vi "ABR-Analyze.vi"(0 "Neural (uV)":dbl[](array[numeric]), 2 "Runtime":T1, 5 "microphonic (uV)":dbl[](array[numeric]), 7 "Averaging data":cluster{i32, i32}, 9 "Normalize individual?":bool, 11 "error in":errorcluster, 12 "Analysis":T3, 13 "Graphs":T2) -> (4 "spread value":dbl, 14 "Analysis out":T3, 15 "error out":errorcluster)   [LabVIEW 2020]
uses:
  TypeDefs/ABR-Analysis State.ctl
  Threshold Estimation VIs/ABR3-Threshold Estimation Result.ctl
  TypeDefs/ABR3-Graph Controls.ctl
  TypeDefs/ABR-Runtime Data.ctl
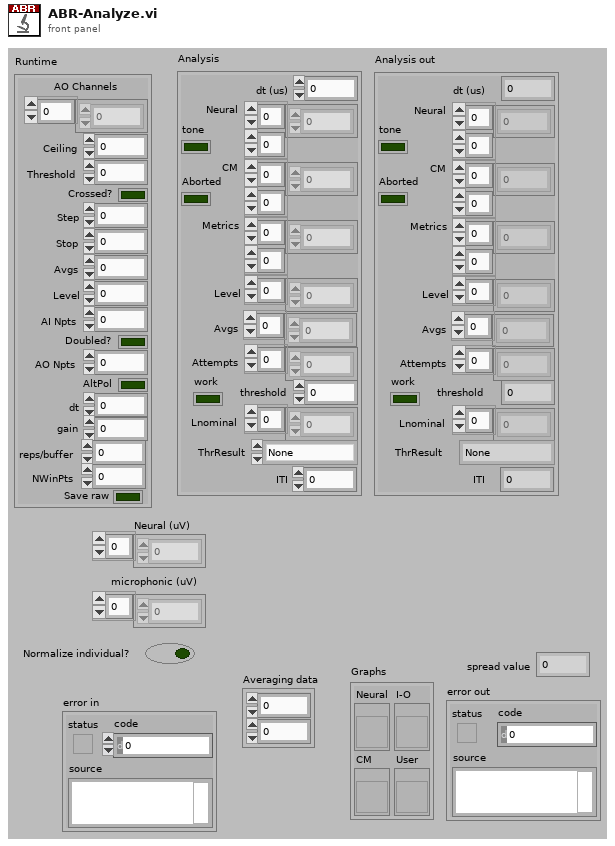
[diagram p1: front panel]
types:
  T1 = typedef "ABR-Runtime Data.ctl" = cluster{"AO Channels":i32[], "Ceiling":dbl, "Threshold":dbl, "Crossed?":bool, "Step":dbl, "Stop":i32, "Avgs":i32, "Level":dbl, "AI Npts":i32, "Doubled?":bool, "AO Npts":i32, "AltPol":bool, "dt":dbl, "gain":dbl, "reps/buffer":i32, "NWinPts":i32, "Save raw":bool}
  T2 = typedef "ABR3-Graph Controls.ctl" = cluster{"I-O":refnum<vi>, "Neural":refnum<vi>, "CM":refnum<vi>, "User":refnum<vi>}
  T3 = typedef "ABR-Analysis State.ctl" = cluster{"dt (us)":dbl, "Neural":dbl[][], "CM":dbl[][], "Metrics":dbl[][], "Level":dbl[], "Avgs":i32[], "Attempts":i32[], "Aborted":bool, "threshold":dbl, "Lnominal":dbl[], "tone":bool, "work":bool, "ThrResult":T4, "ITI":dbl}
  T4 = typedef "ABR3-Threshold Estimation Result.ctl" = enum16{"None", "Power", "Sigmoid", "Power (noisy)", "Suprathreshold", "Invalid"}
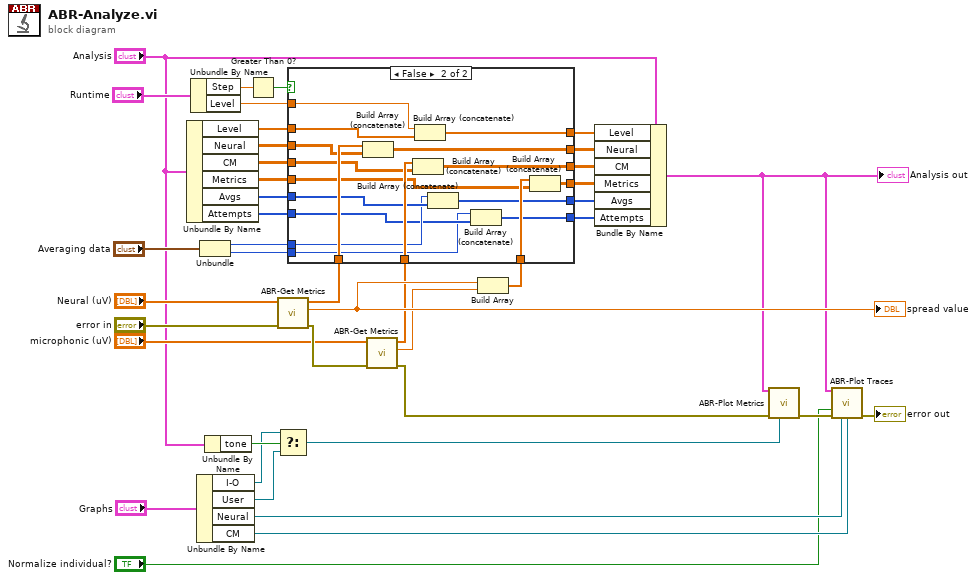
[diagram p0: block diagram]
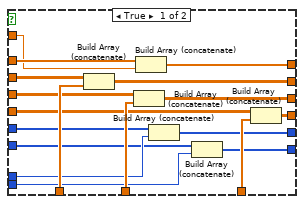
[diagram p2: hidden frame]
diagram:
  n1 = Unbundle By Name("Analysis") -> ("Level"=w27:dbl[], "Neural"=w35:dbl[][], "CM"=w34:dbl[][], "Metrics"=w33:dbl[][], "Avgs"=w18:i32[], "Attempts"=w14:i32[])
  n2 = Unbundle By Name("Runtime") -> ("Step"=w2:dbl, "Level"=w25:dbl)
  n3 = Unbundle By Name("Graphs") -> ("I-O"=w5:refnum<vi>, "User"=w4:refnum<vi>, "Neural"=w21:refnum<vi>, "CM"=w20:refnum<vi>)
  n4 = Unbundle("Averaging data") -> (w16:i32, w12:i32)
  n5 = Unbundle By Name("Analysis") -> ("tone"=w6:bool)
  n6 = Greater Than 0?(x=w2) -> (x > 0?=w1:bool)
  n7 = call "ABR-Get Metrics.vi"("error in (no error)"="error in", "Data in"="Neural (uV)") -> ("error out"=w29:errorcluster, "spread value"=w41:dbl, "Data out"=w39:dbl[])  [unwired: 7 in]
  "spread value" <- w41
  n8 = Select(t=w5, s=w6, f=w4) -> (s? t:f=w3:refnum<vi>)
  n9 = call "ABR-Get Metrics.vi"("error in (no error)"=w29, "Data in"="microphonic (uV)") -> ("error out"=w11:errorcluster, "spread value"=w37:dbl, "Data out"=w38:dbl[])  [unwired: 7 in]
  n10 = Build Array(w41, w37) -> (w40:dbl[])
  n11 = case shown="False" w1 {
    tunnel: w40 -> [w59 w77]
    tunnel: w39 -> [w58 w76]
    tunnel: w38 -> [w57 w75]
    tunnel: w35 -> [w56 w74]
    tunnel: w34 -> [w55 w73]
    tunnel: w33 -> [w54 w72]
    tunnel: [w53 w71] -> w32
    tunnel: [w52 w70] -> w31
    tunnel: [w51 w69] -> w30
    tunnel: w27 -> [w50 w68]
    tunnel: [w49 w67] -> w26
    tunnel: w25 -> [w48 w66]
    tunnel: w18 -> [w47 w65]
    tunnel: w16 -> [w46 w64]
    tunnel: [w45 w63] -> w15
    tunnel: w14 -> [w44 w62]
    tunnel: [w43 w61] -> w13
    tunnel: w12 -> [w42 w60]
    frame True {
      n12 = Build Array (concatenate)(w56, w58) -> (w53:dbl[][])
      n13 = Build Array (concatenate)(w55, w57) -> (w52:dbl[][])
      n14 = Build Array (concatenate)(w50, w48) -> (w49:dbl[])
      n15 = Build Array (concatenate)(w47, w46) -> (w45:i32[])
      n16 = Build Array (concatenate)(w44, w42) -> (w43:i32[])
      n17 = Build Array (concatenate)(w54, w59) -> (w51:dbl[][])
    }
    frame False {
      n18 = Build Array (concatenate)(w76, w74) -> (w71:dbl[][])
      n19 = Build Array (concatenate)(w75, w73) -> (w70:dbl[][])
      n20 = Build Array (concatenate)(w66, w68) -> (w67:dbl[])
      n21 = Build Array (concatenate)(w64, w65) -> (w63:i32[])
      n22 = Build Array (concatenate)(w60, w62) -> (w61:i32[])
      n23 = Build Array (concatenate)(w77, w72) -> (w69:dbl[][])
    }
  }
  n24 = Bundle By Name(cluster="Analysis", "Level"=w26, "Neural"=w32, "CM"=w31, "Metrics"=w30, "Avgs"=w15, "Attempts"=w13) -> (w8:T3)
  "Analysis out" <- w8
  n25 = call "ABR-Plot Metrics.vi"("Analysis"=w8, "error in (no error)"=w11, "I-O"=w3) -> ("error out"=w23:errorcluster)  [unwired: 12 in]
  n26 = call "ABR-Plot Traces.vi"("Analysis"=w8, "Normalize individual?"="Normalize individual?", "error in (no error)"=w23, "Neural Ref"=w21, "CM Ref"=w20) -> ("error out"=→"error out":errorcluster)  [unwired: 10 in]
